vi "Write EventLoggerDVR.vi"(8 "error in (no error)":errorcluster, 10 "EventLoggerDVR":T1, 11 "EventLogger in":refnum<class "EventLogger.lvclass">) -> (0 "error out":errorcluster, 3 "EventLogger out":refnum<class "EventLogger.lvclass">)   [LabVIEW 2015, in "EventLogger.lvclass"]
uses:
  EventLogger.lvclass
  Controls/EventLoggerDVR--DVR.ctl
  EventLogger.lvclass/EventLogger.ctl
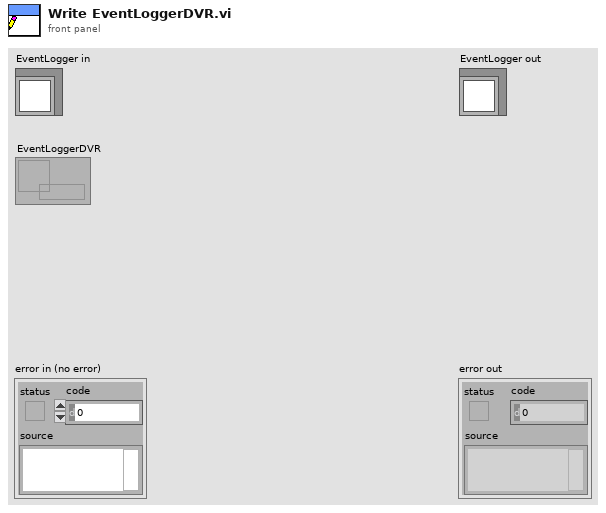
[diagram p1: front panel]
types:
  T1 = typedef "EventLoggerDVR--DVR.ctl" = refnum<data-value>
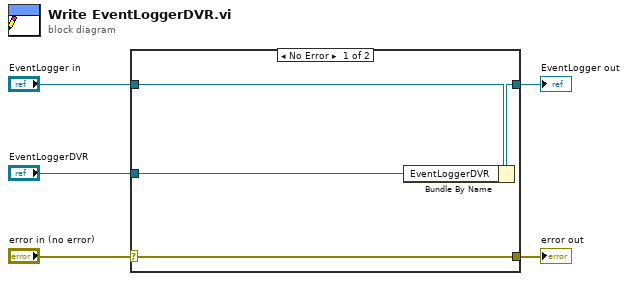
[diagram p0: block diagram]
diagram:
  n1 = case shown="No Error" "error in (no error)" {
    selector: "error in (no error)" -> [w9 w10]
    tunnel: [w9 w10] -> w4
    tunnel: [w7 w11] -> w2
    tunnel: "EventLogger in" -> [w8 w11]
    tunnel: "EventLoggerDVR" -> [w6 _]
    frame No Error {
      n2 = Bundle By Name(cluster=w8, "EventLoggerDVR"=w6) -> (w7:refnum<class "EventLogger.lvclass">)
    }
    frame Error {
    }
  }
  "error out" <- w4
  "EventLogger out" <- w2
